vi "Read VeriSTAND Channel Info.vi"(8 "error in (no error)":errorcluster, 11 "ChannelVS in":refnum<class "ChannelVS.lvclass">) -> (0 "error out":errorcluster, 1 "VeriSTAND Reference":T1=18446744073709551615 format="%.0x", 2 "Exist in VeriSTAND":bool, 3 "ChannelVS out":refnum<class "ChannelVS.lvclass">)   [LabVIEW 2017, in "Shared Variables CD 2.0 Configuration.lvlib" / "ChannelVS.lvclass"]
uses:
  ChannelVS.lvclass
  <vilib>/NI Veristand/Custom Device API/Custom Device Item Ref.ctl
  ChannelVS.lvclass/ChannelVS.ctl
  <vilib>/NI VeriStand/Custom Device API/Custom Device API.lvlib
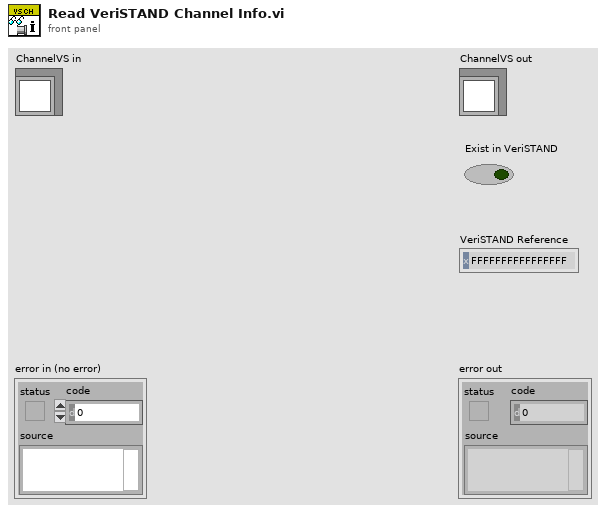
[diagram p1: front panel]
types:
  T1 = typedef "Custom Device API.lvlib/Custom Device Item Ref.ctl" = u64
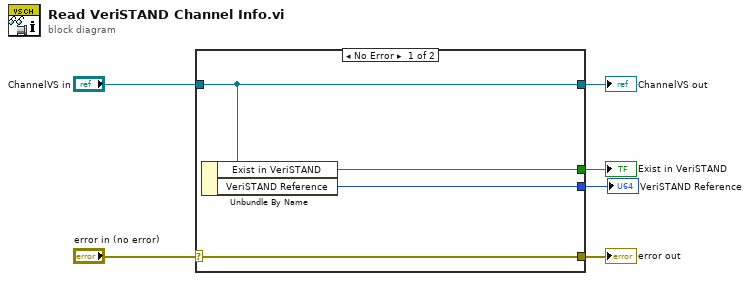
[diagram p0: block diagram]
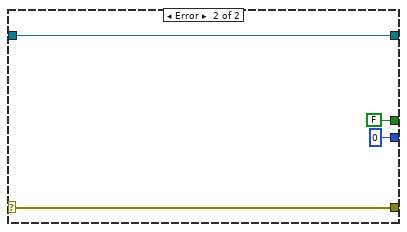
[diagram p2: hidden frame]
diagram:
  n1 = case shown="No Error" "error in (no error)" {
    selector: "error in (no error)" -> [w10 w13]
    tunnel: [w10 w13] -> w5
    tunnel: [w9 w14] -> w3
    tunnel: "ChannelVS in" -> [w9 w14]
    tunnel: [w8 FALSE ("Exist in VeriSTAND")] -> w2
    tunnel: [w7 T1 0 ("VeriSTAND Reference")] -> w1
    frame No Error {
      n2 = Unbundle By Name(w9) -> ("Exist in VeriSTAND"=w8:bool, "VeriSTAND Reference"=w7:T1)
    }
    frame Error {
    }
  }
  "error out" <- w5
  "ChannelVS out" <- w3
  "Exist in VeriSTAND" <- w2
  "VeriSTAND Reference" <- w1
